vi "Get ECAT IOVs.vi"(8 "error in (no error)":errorcluster, 11 "ECAT Slave in":refnum<k21>="ni.var.io://localhost/EtherCAT Master/Device") -> (0 "error IO":errorcluster, 1 "All Mods":refnum<k21>[](array[refnum]), 2 "UDV Container":refnum<k21>[](array[refnum]), 3 "ECAT Slave out":refnum<k21>="ni.var.io:/", 5 "ECAT Variablenobjekt":refnum<k21>[](array[refnum]))   [LabVIEW 2016, in "Scan Engine Custom Device.lvlib"]
uses:
  Scan Engine Custom Device.lvlib
  <resource>/objmgr/IndComECAT.rc
  <resource>/objmgr/ni.var.rc
  <resource>/objmgr/cRIO.rc
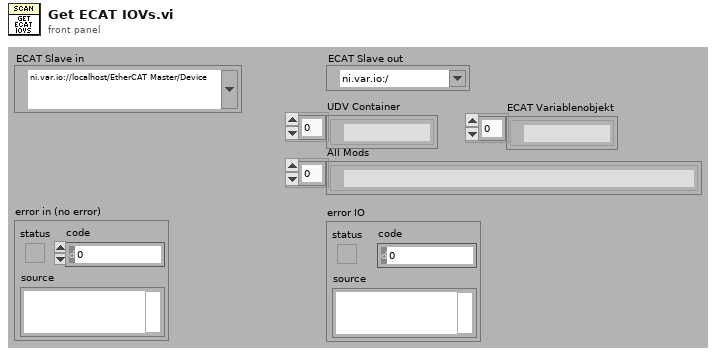
[diagram p1: front panel]
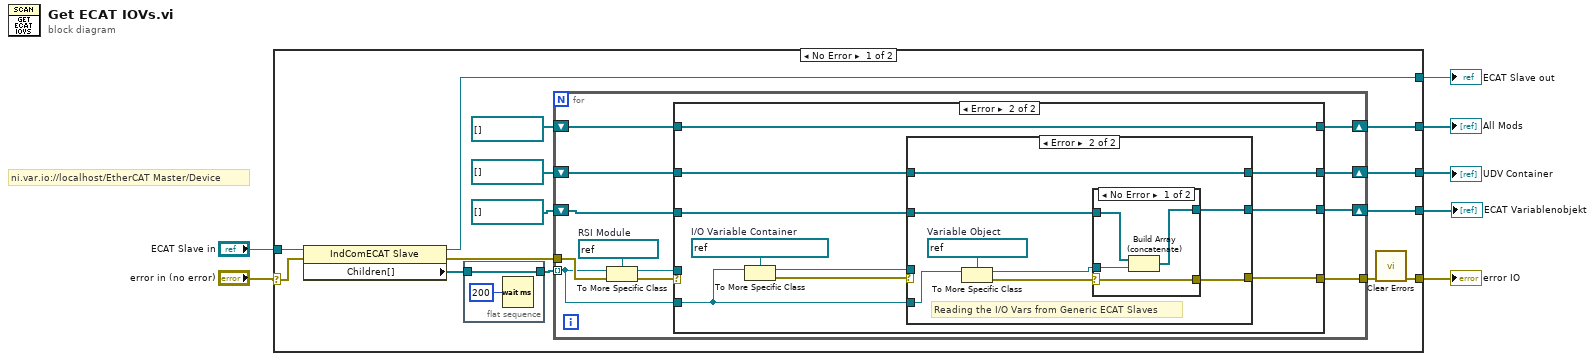
[diagram p0: block diagram]
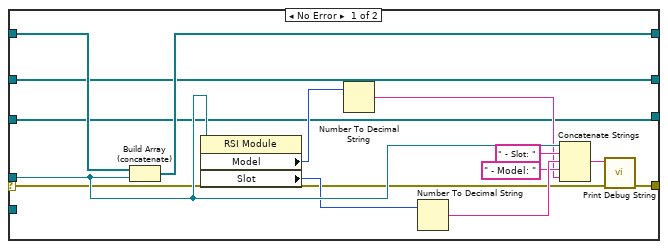
[diagram p2: hidden frame]
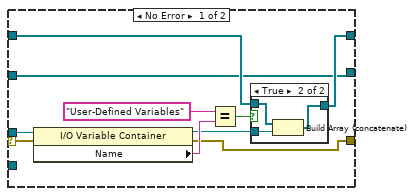
[diagram p3: hidden frame]
diagram:
  # "ni.var.io://localhost/EtherCAT Master/Device"
  n1 = case shown="No Error" "error in (no error)" {
    selector: "error in (no error)" -> [w18 w89]
    tunnel: [w21 w89] -> w7
    tunnel: [w15 _] -> w3
    tunnel: "ECAT Slave in" -> [w20 w88]
    tunnel: [w19 w88] -> w5
    tunnel: [w12 _] -> w2
    tunnel: [w8 _] -> w1
    frame No Error {
      n2 = property class="IndComECAT Slave"(reference=w20, error in=w18) -> (reference out=w19:refnum<k21>, error out=w16:errorcluster, "Children[]"=w11:refnum<k21>[])
      n3 = flat-sequence {
        tunnel: w11 -> [w23]
        tunnel: [w23] -> w10
        frame #0 {
          n4 = Wait (ms)(milliseconds to wait=u32 200) -> ()  [unwired: 1 out]
        }
      }
      n5 = for {
        tunnel: w10 -> [w26] mode=indexing
        tunnel: w16 -> [w35]
        shift-right: [w33] -> w15
        shift-left: refnum<k21>[] [] -> [w32]
        tunnel: [w31] -> w14
        shift-right: [w27] -> w12
        shift-left: refnum<k21>[] [] -> [w28]
        shift-right: [w25] -> w8
        shift-left: refnum<k21>[] [] -> [w24]
        w34 = refnum<k21> refnum  # RSI Module
        n6 = To More Specific Class(target class=w34, reference=w26, error in=w35) -> (specific class reference=w29:refnum<k21>, error out=w30:errorcluster)
        n7 = case shown="Error" w30 {
          selector: w30 -> [w38 _]
          tunnel: w29 -> [w46 _]
          tunnel: [w49 w59] -> w33
          tunnel: w32 -> [w48 w59]
          tunnel: [w39 w53] -> w31
          tunnel: w28 -> [w47 w55]
          tunnel: [w47 w54] -> w27
          tunnel: w26 -> [_ w52]
          tunnel: [w36 w51] -> w25
          tunnel: w24 -> [w36 w50]
          frame No Error {
            n8 = Build Array (concatenate)(w48, w46) -> (w49:refnum<k21>[])
            n9 = property class="RSI Module"(reference=w46) -> ("Model"=w45:u32, "Slot"=w44:u32)  [unwired: 1 in, 2 out]
            n10 = Number To Decimal String(number=w45) -> (decimal integer string=w40:string)  [unwired: 1 in]
            n11 = Number To Decimal String(number=w44) -> (decimal integer string=w42:string)  [unwired: 1 in]
            n12 = Concatenate Strings(w46, " - Slot: " ("string"), w42, " - Model: " ("string"), w40) -> (w37:string)
            n13 = call "Print Debug String.vi"("error in"=w38, "String to write"=w37) -> ("error out"=w39:errorcluster)  [unwired: 8 in]
          }
          frame Error {
            w58 = refnum<k21> refnum  # I/O Variable Container
            n14 = To More Specific Class(target class=w58, reference=w52) -> (specific class reference=w56:refnum<k21>, error out=w57:errorcluster)  [unwired: 1 in]
            n15 = case shown="Error" w57 {
              selector: w57 -> [w69 _]
              tunnel: [w63 w81] -> w54
              tunnel: w56 -> [w68 _]
              tunnel: [w62 w77] -> w53
              tunnel: w55 -> [w61 w81]
              tunnel: w52 -> [_ w76]
              tunnel: [w60 w75] -> w51
              tunnel: w50 -> [w60 w74]
              frame No Error {
                n16 = property class="I/O Variable Container"(reference=w68, error in=w69) -> (reference out=w64:refnum<k21>, error out=w62:errorcluster, "Name"=w67:string)
                n17 = Equal?(x="User-Defined Variables", y=w67) -> (x = y?=w65:bool)
                n18 = case shown="True" w65 {
                  tunnel: w64 -> [_ w72]
                  tunnel: w61 -> [w70 w73]
                  tunnel: [w70 w71] -> w63
                  frame False {
                  }
                  frame True {
                    n19 = Build Array (concatenate)(w73, w72) -> (w71:refnum<k21>[])
                  }
                }
              }
              frame Error {
                w78 = refnum<k21> refnum  # Variable Object
                # "Reading the I/O Vars from Generic ECAT Slaves"
                n20 = To More Specific Class(target class=w78, reference=w76) -> (specific class reference=w80:refnum<k21>, error out=w79:errorcluster)  [unwired: 1 in]
                n21 = case shown="No Error" w79 {
                  selector: w79 -> [w82 w87]
                  tunnel: [w85 w86] -> w75
                  tunnel: w80 -> [w84 _]
                  tunnel: w74 -> [w83 w86]
                  tunnel: [w82 w87] -> w77
                  frame No Error {
                    n22 = Build Array (concatenate)(w83, w84) -> (w85:refnum<k21>[])
                  }
                  frame Error {
                  }
                }
              }
            }
          }
        }
      }
      n23 = call <vilib>:"Clear Errors.vi"("error in (no error)"=w14) -> ("error out"=w21:errorcluster)  [unwired: 5 in, 1 out]
    }
    frame Error {
    }
  }
  "error IO" <- w7
  "ECAT Slave out" <- w5
  "All Mods" <- w3
  "UDV Container" <- w2
  "ECAT Variablenobjekt" <- w1
